vi "select_mclamp_channel.vi"(5 "which manipulator":T1(ring), 8 "error in (no error)":errorcluster, 10 "mclamp cluster":T2, 11 "Multiclamp Handle In":u32=722860) -> (0 "error out":errorcluster, 1 "error":i32, 3 "Multiclamp Handle out":u32=722860)   [LabVIEW 2019]
uses:
  patcherBot_software_all/patcherBot_Software/patcherBot/AxMultiClampMsg.dll
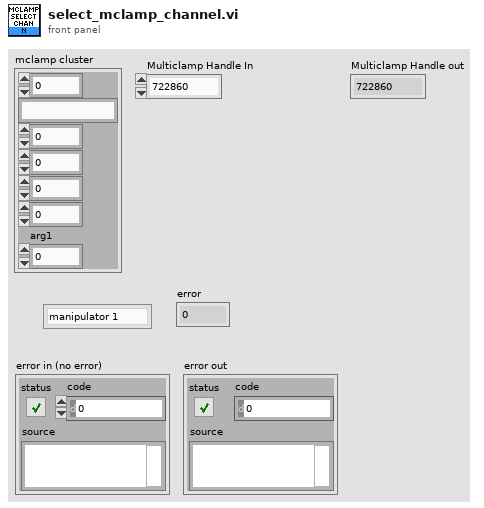
[diagram p1: front panel]
types:
  T1 = enum16{"manipulator 1", "manipulator 2", "manipulator 3", "manipulator 4"}
  T2 = cluster{u32, string, i32, u32, u32, u32, "arg1":i32}
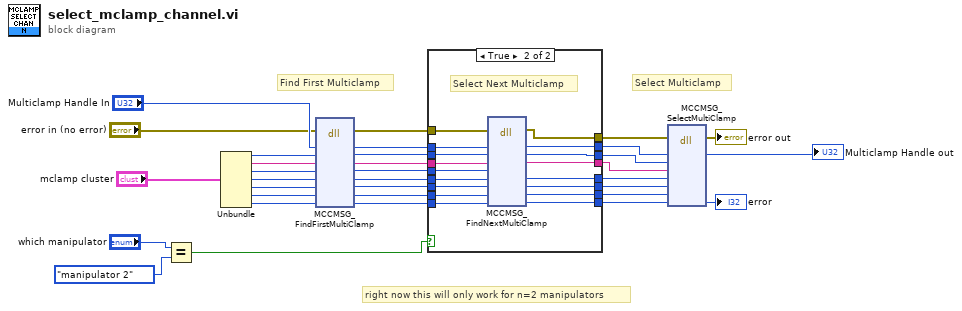
[diagram p0: block diagram]
diagram:
  # "right now this will only work for n=2 manipulators"
  # "Select Multiclamp"
  # "Find First Multiclamp"
  n1 = Equal?(x="which manipulator", y=T1."manipulator 2" ("which manipulator")) -> (x = y?=w14:bool)
  n2 = Unbundle("mclamp cluster") -> (w31:u32, w30:string, w29:i32, w28:u32, w27:u32, w26:u32, "arg1"=w25:i32)
  n3 = dll-call lib="C:/Users/might/Dropbox (GaTech)/patcherBot_software_all/patcherBot_Software/patcherBot/AxMultiClampMsg.dll" fn="MCCMSG_FindFirstMultiClamp"(error in="error in (no error)", "handle"="Multiclamp Handle In", "uModel"=w31, "szSerialNum"=w30, "SnumSize"=w29, "uCOMPortID"=w28, "uDeviceID"=w27, "uChannelID"=w26, "error"=w25) -> (error out=w9:errorcluster, "handle"=w15:u32, "uModel"=w16:u32, "szSerialNum"=w17:string, "SnumSize"=w18:i32, "uCOMPortID"=w19:u32, "uDeviceID"=w20:u32, "uChannelID"=w21:u32, "error"=w22:i32)  [unwired: 3 in, 1 out]
  n4 = case shown="True" w14 {
    tunnel: w22 -> [w38 w58]
    tunnel: w21 -> [w37 w57]
    tunnel: w20 -> [w36 w56]
    tunnel: w19 -> [w35 w55]
    tunnel: w18 -> [_ w54]
    tunnel: w17 -> [w39 w53]
    tunnel: w16 -> [w40 w52]
    tunnel: w15 -> [w41 w51]
    tunnel: [w38 w50] -> w13
    tunnel: [w37 w49] -> w12
    tunnel: [w36 w48] -> w11
    tunnel: [w35 w47] -> w10
    tunnel: w9 -> [w34 w46]
    tunnel: [w34 w45] -> w8
    tunnel: [w39 w44] -> w7
    tunnel: [w41 w43] -> w6
    tunnel: [w40 w42] -> w5
    frame False {
    }
    frame True {
      # "Select Next Multiclamp"
      n5 = dll-call lib="C:/Users/might/Dropbox (GaTech)/patcherBot_software_all/patcherBot_Software/patcherBot/AxMultiClampMsg.dll" fn="MCCMSG_FindNextMultiClamp"(error in=w46, "handle"=w51, "uModel"=w52, "szSerialNum"=w53, "SnumSize"=w54, "uCOMPortID"=w55, "uDeviceID"=w56, "uChannelID"=w57, "error"=w58) -> (error out=w45:errorcluster, "handle"=w43:u32, "uModel"=w42:u32, "szSerialNum"=w44:string, "uCOMPortID"=w47:u32, "uDeviceID"=w48:u32, "uChannelID"=w49:u32, "error"=w50:i32)  [unwired: 4 in, 1 out]
    }
  }
  n6 = dll-call lib="C:/Users/might/Dropbox (GaTech)/patcherBot_software_all/patcherBot_Software/patcherBot/AxMultiClampMsg.dll" fn="MCCMSG_SelectMultiClamp"(error in=w8, "handle"=w6, "uModel"=w5, "szSerialNum"=w7, "uCOMPortID"=w10, "uDeviceID"=w11, "uChannelID"=w12, "error"=w13) -> (error out=→"error out":errorcluster, "handle"=→"Multiclamp Handle out":u32, "error"=→"error":i32)  [unwired: 8 in, 1 out]
